vi "GetHWI.vi"(8 "error in (no error)":errorcluster, 11 "DDS in":refnum<class "DDS.lvclass">) -> (0 "error out":errorcluster, 2 "DDS Hardware Image":T1, 3 "DDS out":refnum<class "DDS.lvclass">)   [LabVIEW 2013, in "DDS.lvclass"]
uses:
  DDS.lvclass
  DDS.lvclass/DDS.ctl
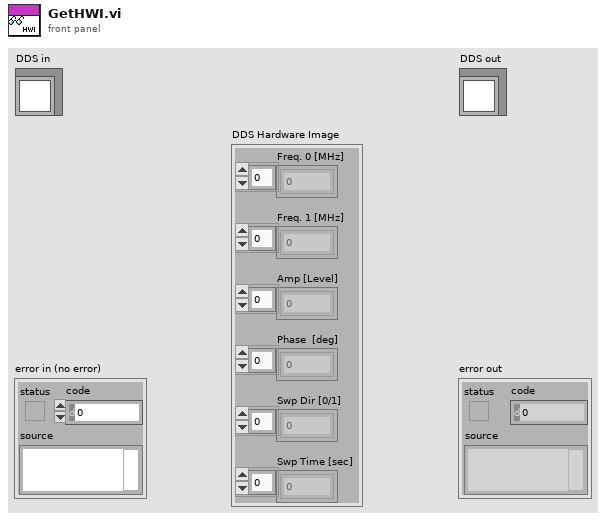
[diagram p1: front panel]
types:
  T1 = cluster{"Freq. 0 [MHz]":dbl[], "Freq. 1 [MHz]":dbl[], "Amp [Level]":dbl[], "Phase  [deg]":dbl[], "Swp Dir [0/1]":i32[], "Swp Time [sec]":dbl[]}
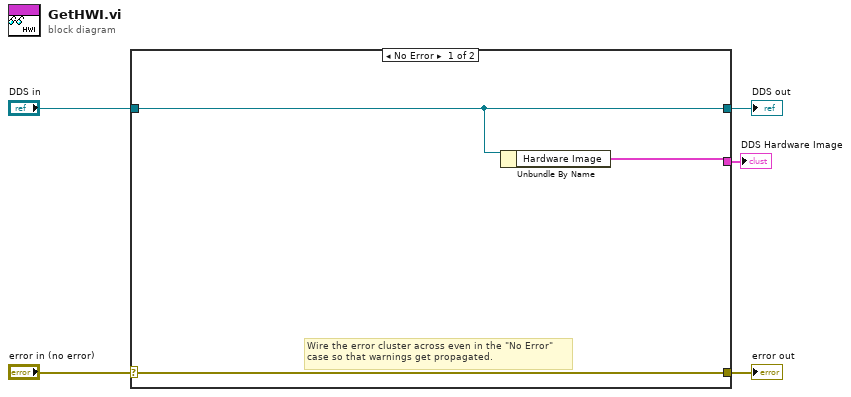
[diagram p0: block diagram]
diagram:
  n1 = case shown="No Error" "error in (no error)" {
    selector: "error in (no error)" -> [w8 w10]
    tunnel: [w8 w10] -> w4
    tunnel: [w7 w9] -> w2
    tunnel: "DDS in" -> [w7 w9]
    tunnel: [w6 _] -> w1
    frame No Error {
      # "Wire the error cluster across even in the \"No Error\"\ncase so that warnings get propagated."
      n2 = Unbundle By Name(w7) -> ("Hardware Image"=w6:T1)
    }
    frame Error {
    }
  }
  "error out" <- w4
  "DDS out" <- w2
  "DDS Hardware Image" <- w1
